vi "Write Content.vi"(8 "Error In":errorcluster, 10 "Content":string, 11 "Text In":refnum<class "Text.lvclass">) -> (0 "Error Out":errorcluster, 3 "Text Out":refnum<class "Text.lvclass">)   [LabVIEW 2018]
uses:
  Text.lvclass
  D:/Users/cfield/Code/Field R&D Services/Mustache/trunk/src/Toolkit/Low-Level/Tokens/Abstract/Abstract.lvclass
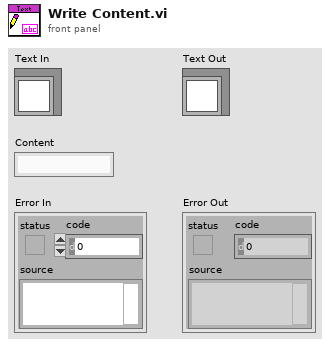
[diagram p1: front panel]
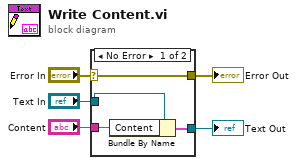
[diagram p0: block diagram]
diagram:
  n1 = case shown="No Error" "Error In" {
    selector: "Error In" -> [w9 w10]
    tunnel: [w9 w10] -> w4
    tunnel: [w7 w11] -> w2
    tunnel: "Text In" -> [w8 w11]
    tunnel: "Content" -> [w6 _]
    frame No Error {
      n2 = Bundle By Name(cluster=w8, "Content"=w6) -> (w7:cluster{})
    }
    frame Error {
    }
  }
  "Error Out" <- w4
  "Text Out" <- w2
